vi "Begin.vi"() -> (0 "error out":errorcluster)   [LabVIEW 2013]
doc: "Called before other user functions, this VI is expected to open initial I/O refnums, load in file data, and do all program initialization. Notice that the <B>error out</B> terminal is simply used for data flow. Wiring it to other structures or subVIs ensures that this VI runs first."
uses:
  <vilib>/Rock Robotics/SystemInterfaces/DIO/FPGA_DIOPWMChannel.ctl
  <vilib>/Rock Robotics/WPI/SafetyOutput/WPI_SafetyOutputConfigMenu.ctl
  <vilib>/Rock Robotics/WPI/DriverStation/WPI_DriverStationRobotMode2.ctl
  <vilib>/Rock Robotics/WPI/Joystick/WPI_JoystickDeviceEnum.ctl
  <vilib>/Rock Robotics/SystemInterfaces/DIO/FPGA_DIORelayChannel.ctl
  <vilib>/Rock Robotics/SystemInterfaces/DIO/FPGA_DIOChannel.ctl
  <vilib>/Rock Robotics/SystemInterfaces/Typedef/FPGA_TypedefDigitalModule.ctl
  DriveAction.ctl
  <vilib>/Rock Robotics/WPI/RobotDrive/WPI_RobotDriveOpen2MotorWithTalon.vi
  Robot Global Data.vi
  OutputError.vi
  OutputErrors.vi
  <vilib>/Rock Robotics/WPI/Compressor/WPI_CompressorGetSetRefNum.vi
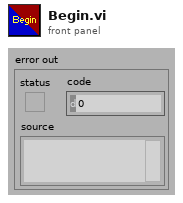
[diagram p1: front panel]
types:
  T1 = typedef "DriveAction.ctl" = enum16{"Init", "LinearDrive", "SetValue", "Disable"}
  T2 = typedef "FPGA_TypedefDigitalModule.ctl" = enum16{"Digital Module 1", "Digital Module 2"}
  T3 = typedef "FPGA_DIOChannel.ctl" = enum8{"DIO 1", "DIO 2", "DIO 3", "DIO 4", "DIO 5", "DIO 6", "DIO 7", "DIO 8", "DIO 9", "DIO 10", "DIO 11", "DIO 12", "DIO 13", "DIO 14", "Invalid"}
  T4 = typedef "FPGA_DIORelayChannel.ctl" = enum8{"Relay 1", "Relay 2", "Relay 3", "Relay 4", "Relay 5", "Relay 6", "Relay 7", "Relay 8", "Invalid"}
  T5 = typedef "WPI_JoystickDeviceEnum.ctl" = enum16{"USB 1", "USB 2", "USB 3", "USB 4", "Kinect 1", "Kinect 2"}
  T6 = typedef "WPI_DriverStationRobotMode2.ctl" = enum16{"Autonomous Disabled", "Autonomous Enabled", "Teleop Disabled", "Teleop Enabled", "Timeout", "Finish", "Test Disabled", "Test Enabled"}
  T7 = typedef "WPI_SafetyOutputConfigMenu.ctl" = enum16{"Enable", "Disable"}
  T8 = typedef "FPGA_DIOPWMChannel.ctl" = enum8{"PWM 1", "PWM 2", "PWM 3", "PWM 4", "PWM 5", "PWM 6", "PWM 7", "PWM 8", "PWM 9", "PWM 10", "Invalid"}
  T9 = typedef "WPI_JoystickDevRef.ctl" = cluster{"Device":T5}
  T10 = typedef "WPI_RobotDriveDevRef.ctl" = cluster{"DevStatus":errorcluster, "Motors[]":T11[], "Square Inputs":bool, "Max Output":dbl, "Isochronous":bool}
  T11 = typedef "WPI_MotorControlDeviceRef.ctl" = cluster{"DeviceStatus":errorcluster, "Type":enum16{"PWM", "CAN"}, "PWM":cluster{"Digital Module":T2, "PWM Channel":T8, "DeadBand":T12}, "CAN":cluster{"Device Number":u8, "Control Mode":T13, "Semaphore":T14, "Max Vout":dbl}, "Invert":bool, "TransformRef":T15, "InvTransformRef":T15}
  T12 = typedef "WPI_PWMDeadband.ctl" = cluster{"Name":string, "maxPositivePwm":i32, "minPositivePwm":i32, "centerPwm":i32, "maxNegativePwm":i32, "minNegativePwm":i32, "angularRange":u16}
  T13 = typedef "WPI_CANJaguar_ControlMode.ctl" = enum8{"Percent VBus", "Current", "Speed", "Position", "Voltage"}
  T14 = typedef "Semaphore RefNum" = refnum<k1>
  T15 = typedef "WPI_PWMTransform_ConPane.ctl" = refnum<vi>
  T16 = typedef "WPI_CompressorDevRef.ctl" = cluster{"DevStatus":errorcluster, "DigitalInputDevRef":T17, "RelayDevRef":T18}
  T17 = typedef "WPI_DigitalInputDevRef.ctl" = cluster{"DevStatus":errorcluster, "DIO Channel":T3, "Digital Module":T2}
  T18 = typedef "WPI_RelayDevRef.ctl" = cluster{"DevStatus":errorcluster, "Relay Channel":T4, "Digital Module":T2, "Relay Direction":T19}
  T19 = typedef "WPI_RelayDirection.ctl" = enum16{"Both directions", "Forward only", "Reverse only"}
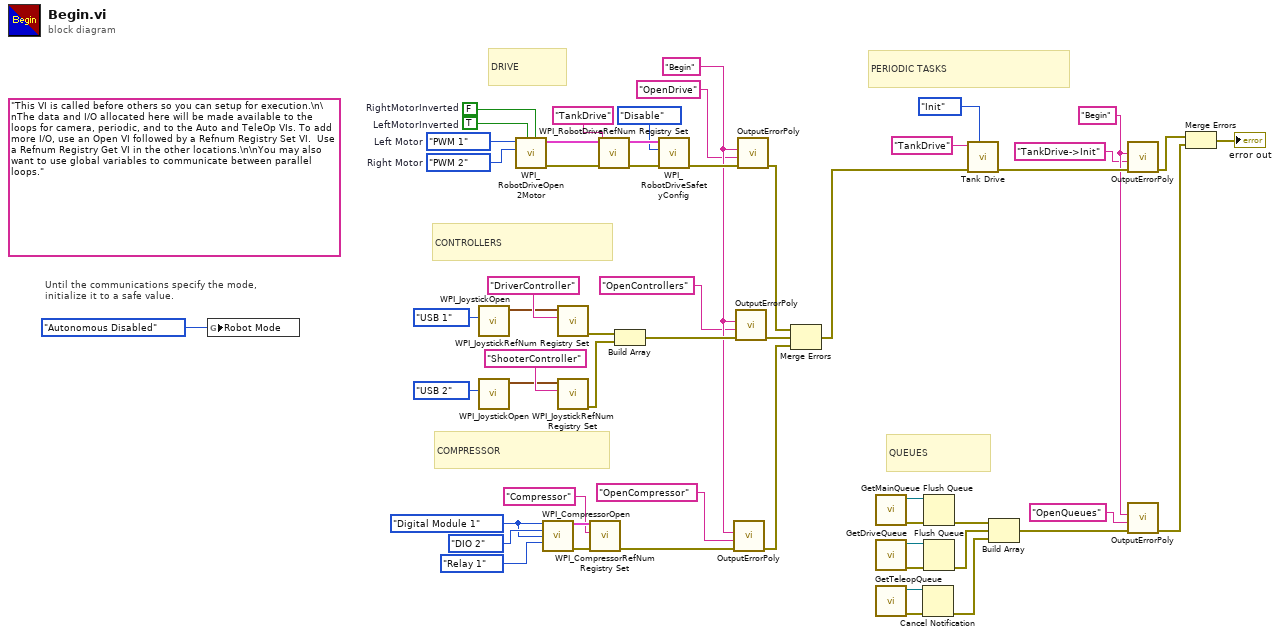
[diagram p0: block diagram]
diagram:
  w10 = "Begin" ("Calling VI")
  w20 = "Begin" ("Calling VI")
  w29 = FPGA_TypedefDigitalModule."Digital Module 1" ("Pressure Switch\nand Relay Module")
  (unwired) "This VI is called before others so you can setup for execution.\n\nThe data and I/O allocated here will be made available to the loops for camera, periodic, and to the Auto and TeleOp VIs. To add more I/O, use an Open VI followed by a Refnum Registry Set VI.  Use a Refnum Registry Get VI in the other locations.\n\nYou may also want to use global variables to communicate between parallel loops."
  w49 = FPGA_DIOPWMChannel."PWM 2"  # Right Motor
  w50 = FPGA_DIOPWMChannel."PWM 1"  # Left Motor
  w54 = TRUE  # LeftMotorInverted
  w55 = FALSE  # RightMotorInverted
  # "PERIODIC TASKS"
  # "QUEUES"
  # "COMPRESSOR"
  # "CONTROLLERS"
  # "DRIVE"
  # "Until the communications specify the mode,\ninitialize it to a safe value."
  n1 = global write "Robot Global Data.vi" "Robot Mode"(WPI_DriverStationRobotMode2."Autonomous Disabled" ("Robot Mode")) -> ()
  n2 = call <vilib>:"WPI_JoystickOpen.vi"("JoystickDevice"=WPI_JoystickDeviceEnum."USB 1") -> ("JoystickDevRef"=w44:T9)  [unwired: 10 in]
  n3 = call <vilib>:"WPI_JoystickOpen.vi"("JoystickDevice"=WPI_JoystickDeviceEnum."USB 2") -> ("JoystickDevRef"=w40:T9)  [unwired: 10 in]
  n4 = call-poly <vilib>:"WPI_RobotDriveOpen2Motor.vi"("Right Motor Inverted"=w55, "Left Motor Inverted"=w54, "Right Motor"=w49, "Left Motor"=w50) -> ("error out"=w51:errorcluster, "RobotDriveDevRef"=w53:T10)  [unwired: 1 in, 5 out]
  n5 = call <vilib>:"WPI_CompressorOpen.vi"("Pressure Switch Digital Module (Module 1)"=w29, "Pressure Switch DIO Channel"=FPGA_DIOChannel."DIO 2" ("Pressure Switch Channel"), "Relay Digital Module (Module 1)"=w29, "Relay Channel"=FPGA_DIORelayChannel."Relay 1") -> ("CompressorDevRef"=w33:T16, "error out"=w31:errorcluster)  [unwired: 1 in, 9 out]
  n6 = call <vilib>:"WPI_JoystickRefNum Registry Set.vi"("refnum name"="DriverController", "JoystickDevRef"=w44) -> ("error out"=w25:errorcluster)  [unwired: 8 in, 1 out]
  n7 = call <vilib>:"WPI_JoystickRefNum Registry Set.vi"("refnum name"="ShooterController", "JoystickDevRef"=w40) -> ("error out"=w24:errorcluster)  [unwired: 8 in, 1 out]
  n8 = call <vilib>:"WPI_CompressorRefNum Registry Set.vi"("error in (no error)"=w31, "refnum name"="Compressor", "CompressorDevRef"=w33) -> ("error out"=w21:errorcluster)  [unwired: 7 in, 1 out]
  n9 = call <vilib>:"WPI_RobotDriveRefNum Registry Set.vi"("error in (no error)"=w51, "refnum name"="TankDrive", "RobotDriveDevRef"=w53) -> ("error out"=w42:errorcluster, "RobotDriveDevRef"=w48:T10)  [unwired: 7 out]
  n10 = Build Array(w25, w24) -> (w22:errorcluster[])
  n11 = call <vilib>:"WPI_RobotDriveSafetyConfig.vi"("error in (no error)"=w42, "mode"=WPI_SafetyOutputConfigMenu."Disable", "RobotDriveDevRef"=w48) -> ("error out"=w23:errorcluster)  [unwired: 7 in, 1 out]
  n12 = call-poly "OutputErrorPoly.vi"("error in (no error)"=w21, "Causing VI"="OpenCompressor", "Calling VI"=w20) -> ("error out"=w3:errorcluster)  [unwired: 8 in]
  n13 = call-poly "OutputErrorPoly.vi"("errors in"=w22, "Causing VI"="OpenControllers", "Calling VI"=w20) -> ("error out"=w4:errorcluster)  [unwired: 8 in]
  n14 = call-poly "OutputErrorPoly.vi"("error in (no error)"=w23, "Causing VI"="OpenDrive", "Calling VI"=w20) -> ("error out"=w2:errorcluster)  [unwired: 8 in]
  n15 = Merge Errors(w2, w4, w3) -> (w1:errorcluster)
  n16 = call "GetMainQueue.vi"() -> ("error out"=w38:errorcluster, "queue out"=w37:refnum<queue>)  [unwired: 10 in]
  n17 = call "GetDriveQueue.vi"() -> ("error out"=w36:errorcluster, "queue out"=w35:refnum<queue>)  [unwired: 10 in]
  n18 = call "GetTeleopQueue.vi"() -> ("error out"=w28:errorcluster, "notifier out"=w27:refnum<notifier>)  [unwired: 10 in]
  n19 = Cancel Notification(0:w27, 3:w28) -> (11:w14:errorcluster)  [unwired: 2 out]
  n20 = Flush Queue(queue=w37, error in (no error)=w38) -> (error out=w16:errorcluster)  [unwired: 2 out]
  n21 = Flush Queue(queue=w35, error in (no error)=w36) -> (error out=w15:errorcluster)  [unwired: 2 out]
  n22 = call "Tank Drive.vi"("DriveAction"=DriveAction."Init", "error in (no error)"=w1, "MotorName"="TankDrive") -> ("error out"=w12:errorcluster)  [unwired: 8 in]
  n23 = Build Array(w16, w15, w14) -> (w13:errorcluster[])
  n24 = call-poly "OutputErrorPoly.vi"("error in (no error)"=w12, "Causing VI"="TankDrive->Init", "Calling VI"=w10) -> ("error out"=w5:errorcluster)  [unwired: 8 in]
  n25 = call-poly "OutputErrorPoly.vi"("errors in"=w13, "Causing VI"="OpenQueues", "Calling VI"=w10) -> ("error out"=w6:errorcluster)  [unwired: 8 in]
  n26 = Merge Errors(w5, w6) -> (→"error out":errorcluster)
